vi "i2c_synch_op.vi"(8 "error in":errorcluster, 10 "Demux command":T1=enum."wait_hard_trigger", 11 "I2C interface":T2) -> (0 "error out":errorcluster, 1 "Empty Elements Remaining":u32)   [LabVIEW 2014]
uses:
  i2c_interface.ctl
  fpga_reference.ctl
  Common/demux_command.ctl
  <vilib>/Utility/error.llb/Error Cluster From Error Code.vi
  <vilib>/rvi/errors/niLvFpgaAdjustHostInterfaceError.vi
  <vilib>/rvi/interface/nirviMethod/nirviMethod.xnode
  FPGA Bitfiles/i2cmuxdemux.lvbitx
  <vilib>/FPGAPlugInAG/PCIe-7842R/niLvFpga_WriteFifo_PCIe-7842R.vi
  <vilib>/rvi/errors/niLvFpgaMergeErrorWithErrorCode.vi
panel:
  # "Send one of the synchronization commands to the I2C demultiplexer.  These commands control synchronization across all of the busses, so do not have a bus argument.  i2c_wait_trigger.vi should also be used on each bus for proper synchronization."
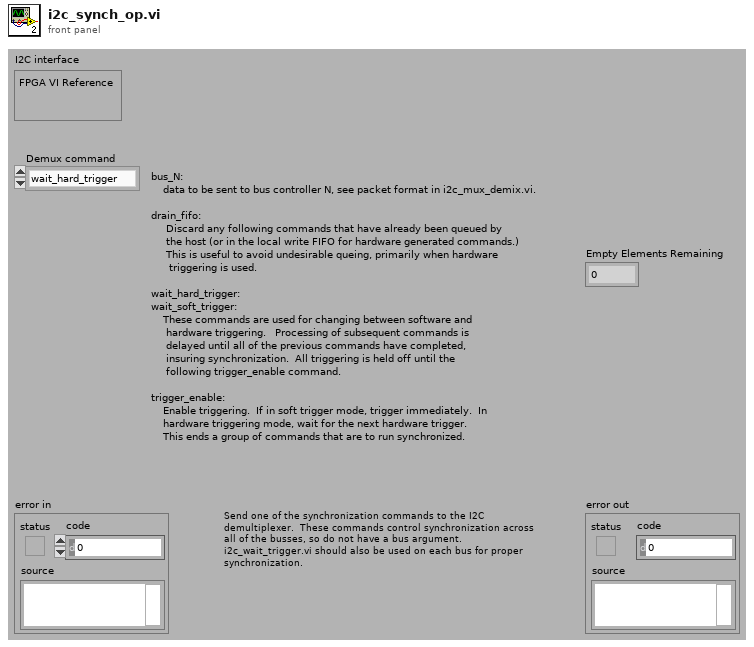
[diagram p1: front panel]
types:
  T1 = typedef "demux_command.ctl" = enum8{"bus_0", "bus_1", "bus_2", "invalid_3", "invalid_4", "drain_fifo", "wait_hard_trigger", "wait_soft_trigger", "trigger_enable"}
  T2 = typedef "i2c_interface.ctl" = cluster{"FPGA VI Reference":T3}
  T3 = typedef "fpga_reference.ctl" = refnum<k20>
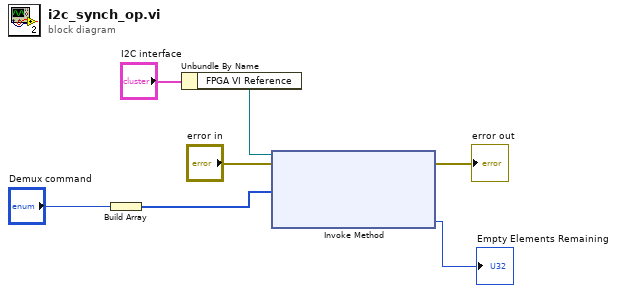
[diagram p0: block diagram]
diagram:
  n1 = Build Array("Demux command") -> (w3:T1[])
  n2 = Unbundle By Name("I2C interface") -> ("FPGA VI Reference"=w6:T3)
  n3 = xnode "Invoke Method"("FPGA VI Reference In"=w6, "error in"="error in", "Data"=w3) -> ("error out"=→"error out":errorcluster, "Empty Elements Remaining"=→"Empty Elements Remaining":u32)  [unwired: 1 in, 1 out]
